vi "stitch interpolated images-ajg.vi"(9 "Calib []":T1, 10 "Array of images to stitch":cluster{u16[][]}[](array[cluster]), 11 "Stitcher in":refnum<class "MagSpecStitcher.lvclass">) -> (2 "stitched array image":u16[][](graph), 3 "Stitcher out":refnum<class "MagSpecStitcher.lvclass">)   [LabVIEW 2013, in "MagSpecStitcher.lvclass"]
uses:
  MagSpecStitcher.lvclass
  image color table presets.ctl
  NI_AALBase.lvlib
  Ramp Pattern by Samples.vi
  CompressAndUpdate(Numeric).vi
  LineoutStats.ctl
  LineoutStatsArray.ctl
panel:
  out "charge vs energy":sgl[](graph)
  out "charge vs angle":sgl[](graph)
  out "x/y":dbl
  out "Energy axis":dbl[](array[numeric])
  out "angle axis":dbl[](array[numeric])
  out "ysize":dbl
  out "size(s)":i32[](array[numeric])
  out "d theta":dbl
  out "length":i32=11
  out "index":i32
  out "img sizes reversed":i32[][](array[numeric])
  out "img pix positions":dbl[](array[numeric])
  out "DeltaE":dbl=1.0
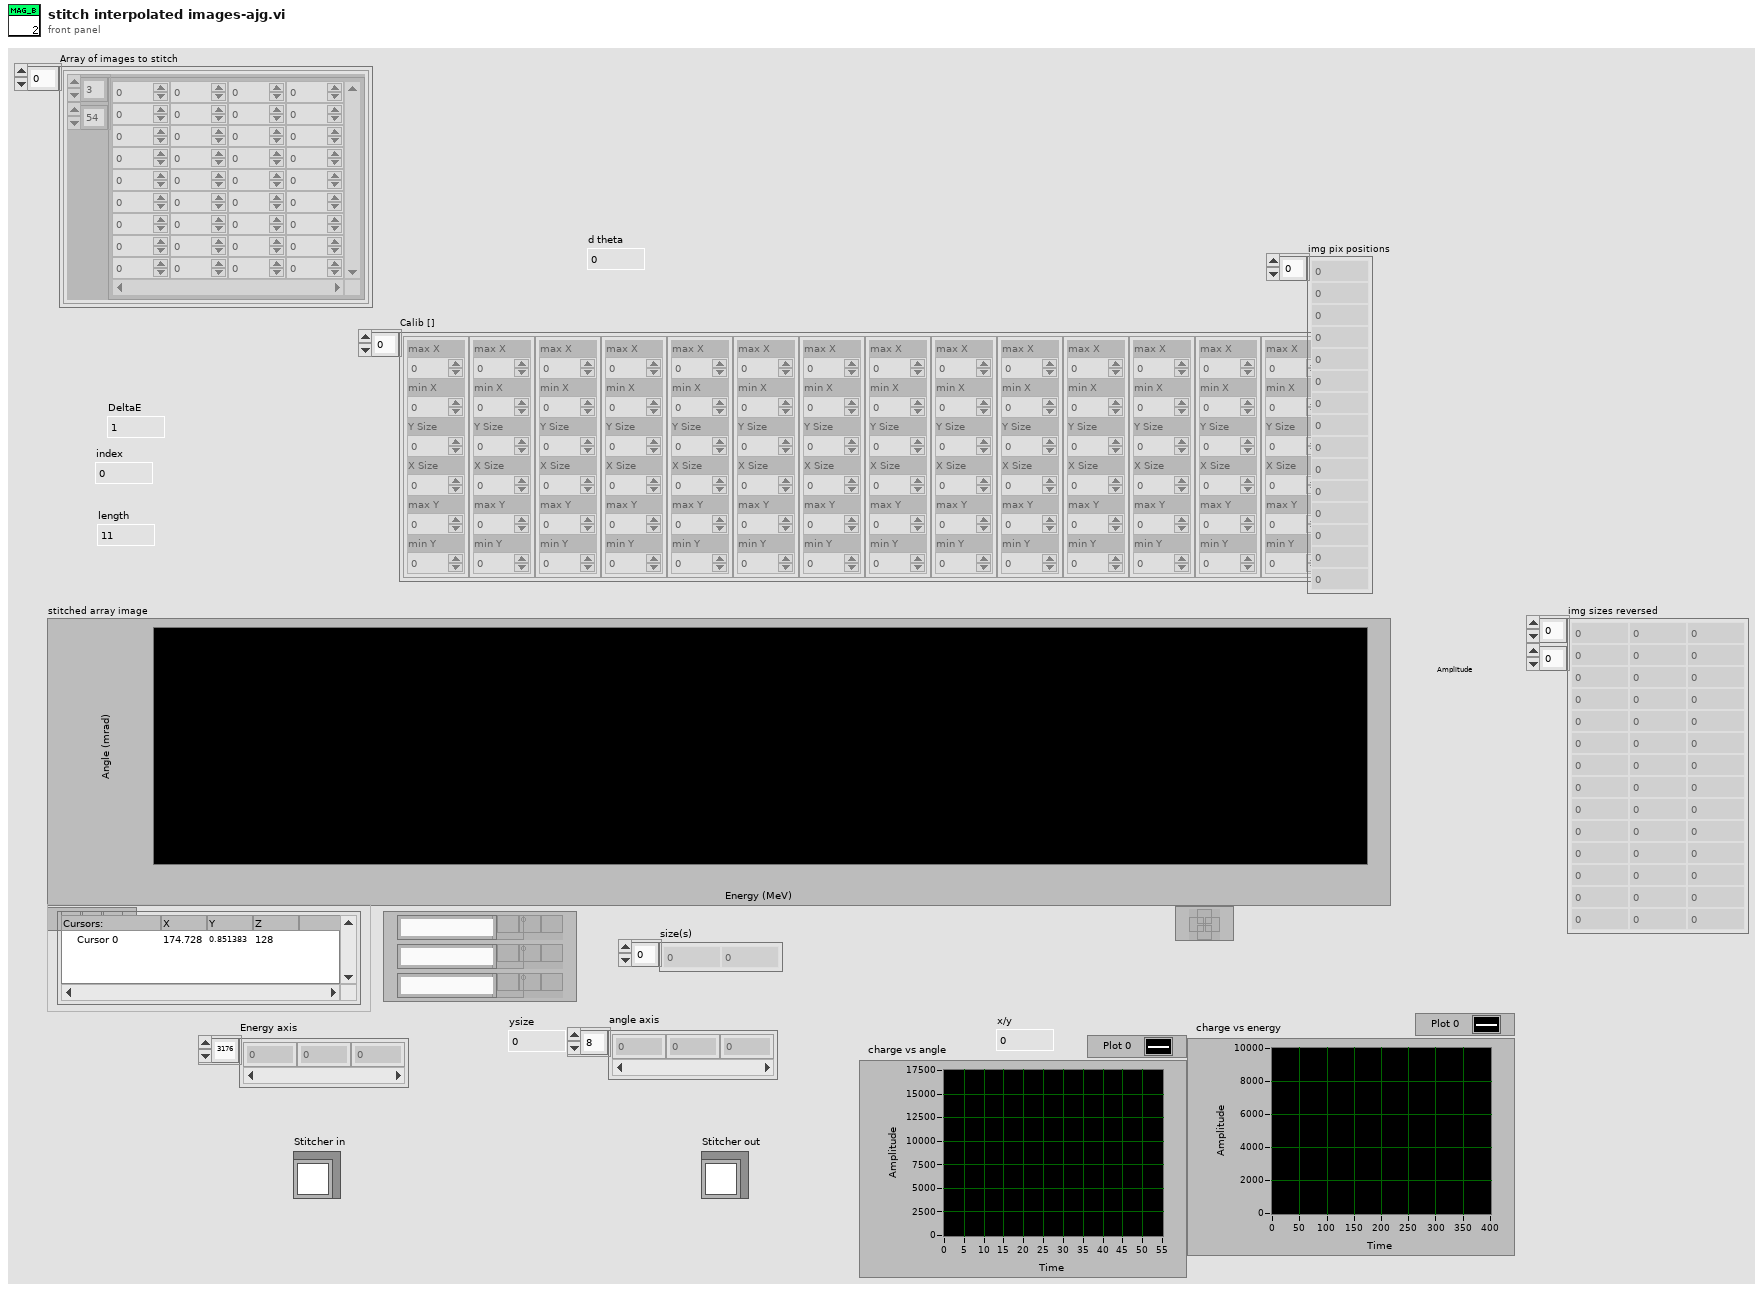
[diagram p1: front panel]
types:
  T1 = typedef "LineoutStatsArray.ctl" = T2[]
  T2 = typedef "LineoutStats.ctl" = cluster{"max X":dbl, "min X":dbl, "Y Size":dbl, "X Size":dbl, "max Y":dbl, "min Y":dbl}
  T3 = typedef "image color table presets.ctl" = enum16{"Greyscale", "Binary", "Gradient", "Rainbow", "Temperature", "enhance low", "blue yellow red", "BYR enhance low", "white blue yellow", "BWR enhance low", "make a new one"}
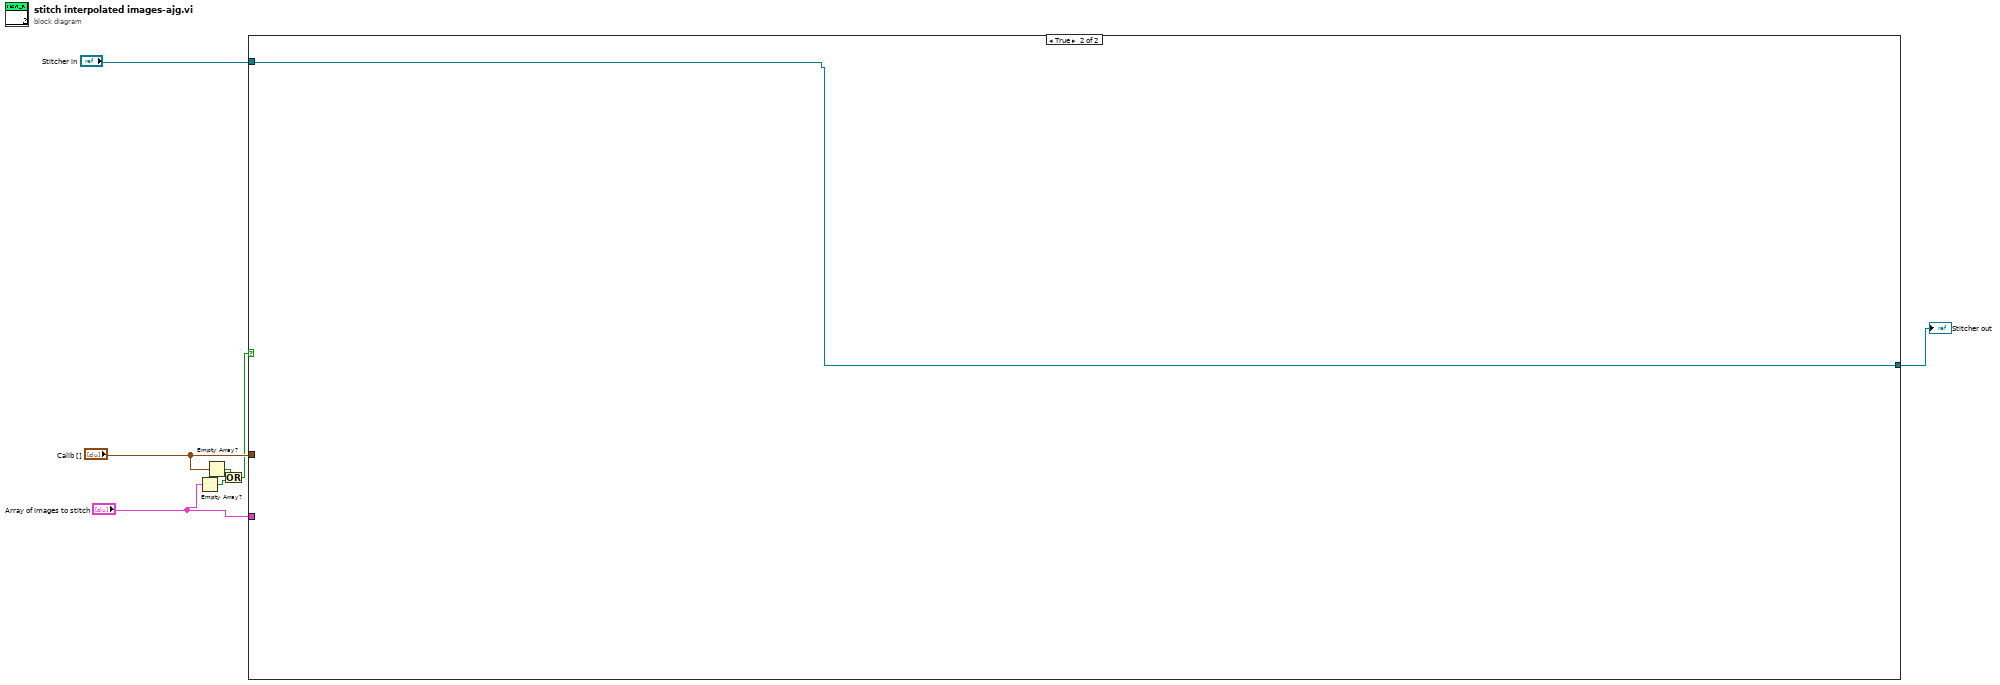
[diagram p0: block diagram]
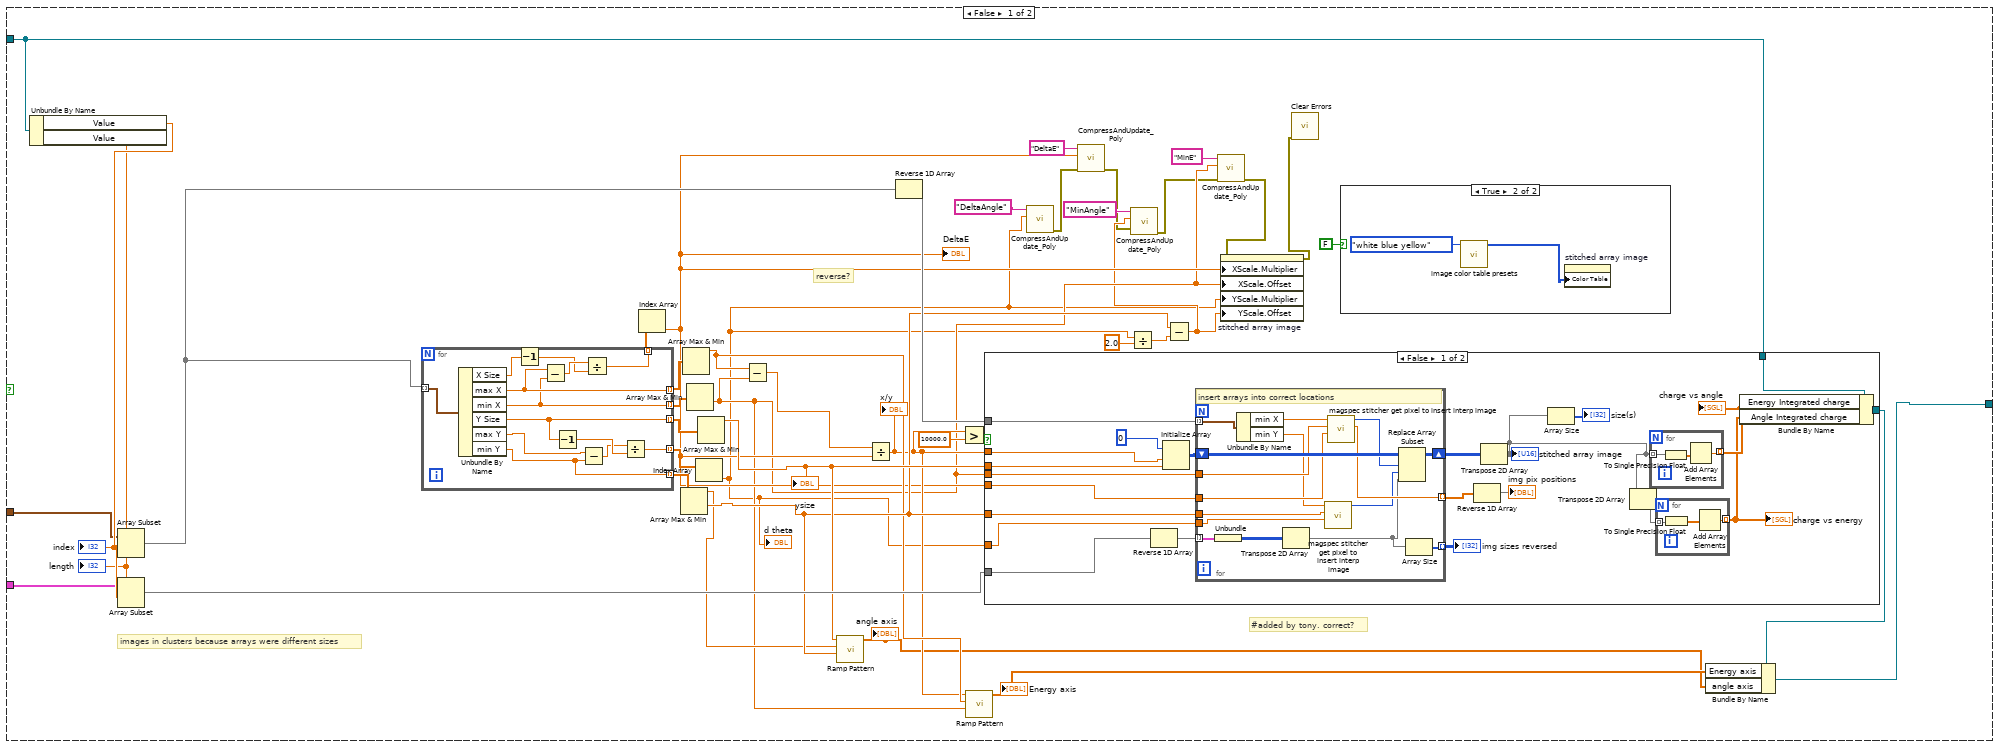
[diagram p2: hidden frame]
diagram:
  n1 = Empty Array?(array="Array of images to stitch") -> (empty?=w3:bool)
  n2 = Empty Array?(array="Calib []") -> (empty?=w4:bool)
  n3 = Or(x=w4, y=w3) -> (x .or. y?=w2:bool)
  n4 = case shown="True" w2 {
    tunnel: "Stitcher in" -> [w16 w110]
    tunnel: "Array of images to stitch" -> [w10 _]
    tunnel: "Calib []" -> [w9 _]
    tunnel: [w8 w110] -> w1
    frame False {
      # "#added by tony. correct?"
      # "reverse?"
      # "images in clusters because arrays were different sizes"
      n5 = Unbundle By Name(w16) -> ("Value"=w15:dbl, "Value"=w14:dbl)
      "index" <- w15
      "length" <- w14
      n6 = Array Subset(array=w9, index=w15, length=w14) -> (w45:T1)
      n7 = Array Subset(array=w10, index=w15, length=w14) -> (w44:cluster{u16[][]}[])
      n8 = for {
        tunnel: w45 -> [w62] mode=indexing
        tunnel: [w61] -> w35 mode=indexing
        tunnel: [w54] -> w32 mode=indexing
        tunnel: [w60] -> w34 mode=indexing
        tunnel: [w58] -> w33 mode=indexing
        tunnel: [w52] -> w31 mode=indexing
        tunnel: [w51] -> w30 mode=indexing
        n9 = Unbundle By Name(w62) -> ("X Size"=w50:dbl, "max X"=w61:dbl, "min X"=w60:dbl, "Y Size"=w54:dbl, "max Y"=w53:dbl, "min Y"=w51:dbl)
        n10 = Decrement(x=w50) -> (x-1=w57:dbl)
        n11 = Subtract(x=w61, y=w60) -> (x-y=w59:dbl)
        n12 = Decrement(x=w54) -> (x-1=w56:dbl)
        n13 = Subtract(x=w53, y=w51) -> (x-y=w55:dbl)
        n14 = Divide(x=w59, y=w57) -> (x/y=w58:dbl)
        n15 = Divide(x=w55, y=w56) -> (x/y=w52:dbl)
      }
      n16 = Index Array(array=w33) -> (element=w29:dbl)  [unwired: 1 in]
      "DeltaE" <- w29
      n17 = Array Max & Min(array=w30) -> (max value=w38:dbl, min value=w39:dbl)  [unwired: 2 out]
      n18 = Array Max & Min(array=w35) -> (max value=w37:dbl)  [unwired: 3 out]
      n19 = Array Max & Min(array=w34) -> (min value=w26:dbl)  [unwired: 3 out]
      n20 = Index Array(array=w31) -> (element=w22:dbl)  [unwired: 1 in]
      "d theta" <- w22
      n21 = Array Max & Min(array=w32) -> (max value=w40:dbl)  [unwired: 3 out]
      "ysize" <- w40
      n22 = Subtract(x=w37, y=w26) -> (x-y=w49:dbl)
      n23 = call-poly "Ramp Pattern.vi"("start"=w39, "end"=w38, "samples"=w40) -> ("Ramp Pattern"=w12:dbl[])  [unwired: 7 in, 1 out]
      "angle axis" <- w12
      n24 = Divide(x=w49, y=w29) -> (x/y=w36:dbl)
      "x/y" <- w36
      n25 = Reverse 1D Array(array=w45) -> (reversed array=w46:T1)
      n26 = Greater?(x=w36, y=10000.0) -> (0:w47:bool)
      n27 = call-poly "Ramp Pattern.vi"("start"=w26, "end"=w37, "samples"=w36) -> ("Ramp Pattern"=w13:dbl[])  [unwired: 7 in, 1 out]
      "Energy axis" <- w13
      n28 = case shown="False" w47 {
        tunnel: w26 -> [w86 _]
        tunnel: w40 -> [w83 _]
        tunnel: w46 -> [w82 _]
        tunnel: w29 -> [w81 _]
        tunnel: w36 -> [w80 _]
        tunnel: w44 -> [w77 _]
        tunnel: w22 -> [w74 _]
        tunnel: w39 -> [w75 _]
        tunnel: w16 -> [w68 w109]
        tunnel: [w65 w109] -> w11
        frame False {
          n29 = Reverse 1D Array(array=w77) -> (reversed array=w85:cluster{u16[][]}[])
          n30 = Initialize Array(u16 0, w80, w83) -> (w84:u16[][])
          n31 = for {
            tunnel: w81 -> [w106]
            shift-right: [w105] -> w71
            shift-left: w84 -> [w108]
            tunnel: w85 -> [w107] mode=indexing
            tunnel: w86 -> [w97]
            tunnel: w82 -> [w103] mode=indexing
            tunnel: [w101] -> w79 mode=indexing
            tunnel: [w99] -> w78 mode=indexing
            tunnel: w75 -> [w95]
            tunnel: w74 -> [w94]
            # "insert arrays into correct locations"
            n32 = Unbundle(w107) -> (w100:u16[][])
            n33 = Unbundle By Name(w103) -> ("min X"=w102:dbl, "min Y"=w96:dbl)
            n34 = Transpose 2D Array(2D array=w100) -> (transposed array=w98:u16[][])
            n35 = call "magspec stitcher get pixel to insert interp image.vi"("Delta"=w94, "min X of all"=w95, "min X of current"=w96) -> ("X pixel to insert into"=w93:i32)  [unwired: 7 in, 1 out]
            n36 = call "magspec stitcher get pixel to insert interp image.vi"("Delta"=w106, "min X of all"=w97, "min X of current"=w102) -> ("x pixel double prec"=w101:dbl, "X pixel to insert into"=w104:i32)  [unwired: 7 in]
            n37 = Replace Array Subset(array=w108, new element=w98, index (row)=w104, index (col)=w93) -> (w105:u16[][])
            n38 = Array Size(array=w98) -> (size(s)=w99:i32[])
          }
          "img sizes reversed" <- w78
          n39 = Reverse 1D Array(array=w79) -> (reversed array=→"img pix positions":dbl[])
          n40 = Transpose 2D Array(2D array=w71) -> (transposed array=w70:u16[][])
          "stitched array image" <- w70
          n41 = Array Size(array=w70) -> (size(s)=→"size(s)":i32[])
          n42 = Transpose 2D Array(2D array=w70) -> (transposed array=w69:u16[][])
          n43 = for {
            tunnel: w70 -> [w91] mode=indexing
            tunnel: [w92] -> w67 mode=indexing
            n44 = To Single Precision Float(number=w91) -> (single precision float=w90:sgl[])
            n45 = Add Array Elements(numeric array=w90) -> (sum=w92:sgl)
          }
          "charge vs angle" <- w67
          n46 = for {
            tunnel: w69 -> [w88] mode=indexing
            tunnel: [w89] -> w66 mode=indexing
            n47 = To Single Precision Float(number=w88) -> (single precision float=w87:sgl[])
            n48 = Add Array Elements(numeric array=w87) -> (sum=w89:sgl)
          }
          "charge vs energy" <- w66
          n49 = Bundle By Name(cluster=w68, "Energy Integrated charge"=w67, "Angle Integrated charge"=w66) -> (w65:refnum<class "MagSpecStitcher.lvclass">)
        }
        frame True {
        }
      }
      n50 = call-poly "CompressAndUpdate_Poly.vi"("Numeric"=w22, "command or variable name"="DeltaAngle") -> ("error out"=w21:errorcluster)  [unwired: 9 in]
      n51 = call-poly "CompressAndUpdate_Poly.vi"("error in"=w21, "Numeric"=w29, "command or variable name"="DeltaE") -> ("error out"=w20:errorcluster)  [unwired: 8 in]
      n52 = Divide(x=w22, y=2.0) -> (x/y=w41:dbl)
      n53 = Subtract(x=w39, y=w41) -> (x-y=w24:dbl)
      n54 = call-poly "CompressAndUpdate_Poly.vi"("error in"=w20, "Numeric"=w24, "command or variable name"="MinAngle") -> ("error out"=w19:errorcluster)  [unwired: 8 in]
      n55 = call-poly "CompressAndUpdate_Poly.vi"("error in"=w19, "Numeric"=w26, "command or variable name"="MinE") -> ("error out"=w18:errorcluster)  [unwired: 8 in]
      n56 = property on="stitched array image" class="IntGraph (strict)"(error in=w18, "XScale.Multiplier"=w29, "XScale.Offset"=w26, "YScale.Multiplier"=w22, "YScale.Offset"=w24) -> (error out=w17:errorcluster)  [unwired: 1 in, 1 out]
      n57 = call "Clear Errors.vi"("error in (no error)"=w17) -> ()  [unwired: 6 in, 1 out]
      n58 = case shown="True" FALSE {
        frame False {
        }
        frame True {
          n59 = call "image color table presets.vi"("Color table"=image_color_table_presets."white blue yellow") -> ("white to yellow color table"=w63:u32[])  [unwired: 9 in, 1 out]
          n60 = property on="stitched array image" class="IntGraph (strict)"("Color Table"=w63) -> ()  [unwired: 2 in, 2 out]
        }
      }
      n61 = Bundle By Name(cluster=w11, "Energy axis"=w13, "angle axis"=w12) -> (w8:refnum<class "MagSpecStitcher.lvclass">)
    }
    frame True {
    }
  }
  "Stitcher out" <- w1
